vi "imp_test_v1.vi"() -> ()   [LabVIEW 2014]
uses:
  <vilib>/LabVIEW Targets/FPGA/cRIO/shared/nicrio_ModuleControls/nicrio_cRIO-9237_DataRatesRing.ctl
  <vilib>/LabVIEW Targets/FPGA/cRIO/shared/nicrio_ModuleControls/nicrio_cRIO-9237_ExcitationVoltageRing.ctl
  <vilib>/rvi/FXPMathLib/FxpSinAndCos/subVIs/nifxpmath_SinAndCos_SimConfig.ctl
  <vilib>/Platform/TimedLoop/XDataNode/timing_clust.ctl
  <vilib>/Platform/TimedLoop/XDataNode/nitl_modes.ctl
  <vilib>/Platform/TimedLoop/XDataNode/wakeup.ctl
  <vilib>/rvi/FXPMathLib/basic elements/FxpIntAccumulator/subVIs/nifxpmath_IntAccumulator_SimConfig.ctl
  <vilib>/rvi/FXPMathLib/FxpSqrt/subVIs/nifxpmath_Sqrt_SimConfig.ctl
  <vilib>/fxp/LVFixedPointOverflowPolicyTypeDef.ctl
  <vilib>/rvi/Emulation/niFpgaGetClockAttributes.vi
  <vilib>/rvi/Emulation/niFpgaSctlEmulationGetInTimedLoop.vi
  <vilib>/rvi/Emulation/niFpgaEmulationReportErrorSimple.vi
  <vilib>/rvi/Emulation/niFpgaProcessEmulError.vi
  <vilib>/rvi/interface/RandomDataEmulation/nirviRandomDataMultiElementFPGAFIFO.vi
  <instcachedir>/0/nirviRandomDataMultiElementFPGAFIFO_AD0CFC12EF974623A9C2E4184BC062B2.lvgen/nirviRandomDataMultiElementFPGAFIFO_AD0CFC12EF974623A9C2E4184BC062B2_023.vi
  <vilib>/rvi/interface/RandomDataEmulation/niFpgaRandomDataHandleErrors.vi
  <vilib>/rvi/Emulation/niFpgaCriticalErrorInLSC.vi
  <vilib>/rvi/eio/common/nirviEmuTemplateMethod_errors.vi
  <vilib>/rvi/FXPMathLib/FxpSinAndCos/simVIs/DllFxpSinAndCosTemp_sub.vi
  <vilib>/rvi/eio/common/nirviEmuTemplatePropertySet_errors.vi
  <vilib>/rvi/Analysis/common/codeGenErrors/XNode/niFpgaXNodeCodeGenErrorHandle.vi
  <vilib>/rvi/FXPMathLib/basic elements/FxpIntAccumulator/simVIs/DllFxpIntAccumulator_sub.vi
  <vilib>/rvi/FXPMathLib/FxpSqrt/simVIs/DllSqrtTemp_sub.vi
  <vilib>/rvi/DataTransferAndStorage/Container/XNode/niFpgaContainer.xnode
  <vilib>/rvi/interface/RandomDataEmulation/nirviRandomDataFpgaMultiElementTemplate.vi
  <vilib>/eio/EIONode/EIONode.xnode
  <vilib>/rvi/FXPMathLib/FxpMul/XNode/nifxpmath_Multiplier.xnode
  <vilib>/rvi/FXPMathLib/FxpSinAndCos/XNode/nifxpmath_SinAndCos.xnode
  <vilib>/rvi/Analysis/measure/butterworth/XNode/niFpgaButterworthFilter.xnode
  <vilib>/rvi/FXPMathLib/FxpSub/XNode/nifxpmath_Sub.xnode
  <vilib>/rvi/FXPMathLib/FxpAdd/XNode/nifxpmath_Add.xnode
  <vilib>/eio/EIOPropertyNode/EIOPropertyNode.xnode
  <vilib>/rvi/Analysis/measure/dc-rms/XNode/niFpgaDC-RMS.xnode
  <vilib>/Platform/TimedLoop/XDataNode/XDataNode.xnode
  <vilib>/rvi/FXPMathLib/basic elements/FxpIntAccumulator/XNode/nifxpmath_IntAccumulator.xnode
  <vilib>/rvi/FXPMathLib/FxpSqrt/XNode/nifxpmath_Sqrt.xnode
  <vilib>/rvi/eio/common/nirviEmuTemplatePropertyGet_errors.vi
  <vilib>/rvi/eio/common/nirviEmuTemplatePropertyGet_noerrors.vi
  <vilib>/rvi/eio/common/nirviEmuTemplatePropertySet_noerrors.vi
  <vilib>/Platform/TimedLoop/XDataNode/XDNodeRunTimeDep.lvlib
  <vilib>/rvi/FXPMathLib/sim/FxpSim.dll
panel:
  in  "ft_d or dt_d2":i16(ring) items=["ft_d", "ft_d2"]
  out "vb":fxp<+/-,38,8>
  out "va":fxp<+/-,38,8>
  out "ft_d2":fxp<+/-,64,59>
  out "Force_r":fxp<+/-,64,42>
  in  "Bv":fxp<+/-,22,8>
  out "D_error_dd":fxp<+/-,64,49>
  out "D_error_d":fxp<+/-,33,10>
  in  "Kv":fxp<+/-,22,8>
  out "D_error":fxp<+/-,64,33>
  out "Dr_sin_dd":fxp<+/-,64,48>
  out "Dr_sin_d":fxp<+/-,64,17>
  out "Sin omega":fxp<+/-,52,9>
  out "Dr_sin":fxp<+/-,39,10>
  in  "Sin offset":fxp<+/-,38,9>
  in  "Sin magnitude":fxp<+/-,22,7>
  out "Time now(s)":fxp<+,52,14>
  in  "Sin wave freq. (Hz)":fxp<+/-,32,6>
  in  "Dr":fxp<+/-,22,7>
  in  "Drive mode":i16(ring) items=["Backward", "Forward"]
  in  "ft_d coeff.":i32[](array[numeric])=[946630756, 63555534]
  out "ft_d":fxp<+/-,36,25>
  out "D_dd":fxp<+/-,36,24>
  in  "D_dd coeff.":i32[](array[numeric])=[946630756, 63555534]
  out "dF_PID":fxp<+/-,36,33>
  in  "dF_PID coeff.":i32[](array[numeric])=[946630756, 63555534]
  out "ft_i":fxp<+/-,34,18>
  out "F_PID":fxp<+/-,51,14>
  in  "f_tolorance":fxp<+,22,6>
  in  "Ki":fxp<+/-,36,9>
  in  "Kd":fxp<+/-,36,9>
  out "f_tilde":fxp<+/-,33,11>
  in  "Kp":fxp<+/-,36,9>
  out "vq_F":fxp<+/-,20,5> format="%.57g"
  out "vd_F":fxp<+/-,20,5>
  in  "dF_add":bool
  out "D_d(mm/s)":fxp<+/-,41,10>
  out "omega(rad/s)":fxp<+/-,20,9>
  in  "Veolcity Estimation":i16(ring) items=["T method", "M_avg method", "M method"]
  in  "Stop motor":bool
  out "D_d(T)":fxp<+/-,41,10>
  out "omega(T)":fxp<+/-,20,9>
  in  "mt0_omega":u32
  out "mt_omega":u32
  out "rad(NrTheta)":fxp<+/-,33,10>
  out "D(mm)":fxp<+/-,32,10>
  out "Encoder Position":i32
  in  "Encoder reset":bool
  in  "Ini coe.":bool
  out "Loop rate (kHz)":fxp<+/-,36,7>
  out "Strain (RMS)":fxp<+,32,44>
  in  "Strain filter coeff.":i32[](array[numeric])=[-850883994, 1909449570, 3794062, -975456236, 2033039520, 4039635]
  out "Force":fxp<+/-,32,10>
  out "Strain":fxp<+/-,42,8>
  out "Fileterd data":fxp<+/-,32,4>
  out "Raw Force":fxp<+/-,32,10>
  in  "S/F coeff":fxp<+/-,41,4>
  out "Raw Strain":fxp<+/-,42,8>
  in  "Reset":bool
  in  "Stop (Strain)":bool
  out "Mod6/AI2":fxp<+/-,32,4>
  in  "Shunt Cal Enable":bool
  in  "Half-Bridge Enable":bool
  in  "Excitation Voltage":T1 items=["2.5 Volts", "3.3 Volts", "5.0 Volts", "10.0 Volts", "External Excitation"]
  in  "Data Rate":T2=1 items=["50.000 kS/s (NI 9237)"=1, "25.000 kS/s (NI 9237)"=2, "16.667 kS/s (NI 9237)"=3, "12.500 kS/s (NI 9237)"=4, "10.000 kS/s (NI 9237)"=5, "8.333 kS/s (NI 9237)"=6, "7.143 kS/s (NI 9237)"=7, "6.250 kS/s (NI 9237)"=8, "5.556 kS/s (NI 9237)"=9, "5.000 kS/s (NI 9237)"=10, "4.545 kS/s (NI 9237)"=11, "4.167 kS/s (NI 9237)"=12, "3.846 kS/s (NI 9237)"=13, "3.571 kS/s (NI 9237)"=14, "3.333 kS/s (NI 9237)"=15, "3.125 kS/s (NI 9237)"=16, "2.941 kS/s (NI 9237)"=17, "2.778 kS/s (NI 9237)"=18, "2.632 kS/s (NI 9237)"=19, "2.500 kS/s (NI 9237)"=20, "2.381 kS/s (NI 9237)"=21, "2.273 kS/s (NI 9237)"=22, "2.174 kS/s (NI 9237)"=23, "2.083 kS/s (NI 9237)"=24, "2.000 kS/s (NI 9237)"=25, "1.923 kS/s (NI 9237)"=26, "1.852 kS/s (NI 9237)"=27, "1.786 kS/s (NI 9237)"=28, "1.724 kS/s (NI 9237)"=29, "1.667 kS/s (NI 9237)"=30, "1.613 kS/s (NI 9237)"=31]
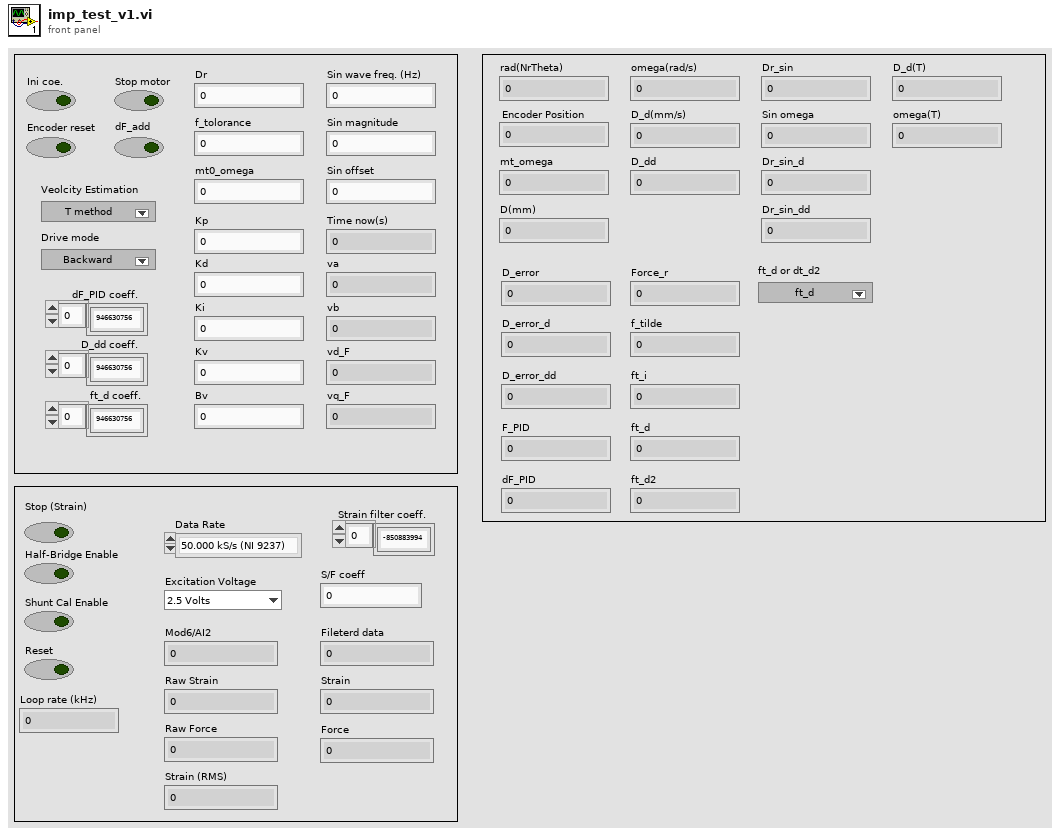
[diagram p1: front panel]
types:
  T1 = typedef "nicrio_cRIO-9237_ExcitationVoltageRing.ctl" = u8
  T2 = typedef "nicrio_cRIO-9237_DataRatesRing.ctl" = u8
  T3 = typedef "XDNodeRunTimeDep.lvlib/timing_clust.ctl" = cluster{"Expected End [f-1]":u64, "Actual End [f-1]":u64, "Finished Late? [f-1]":bool, "Expected End [i-1]":u64, "Actual End [i-1]":u64, "Finished Late? [i-1]":bool, "Expected Start [i]":u64, "Actual Start [i]":u64, "Expected Start [f]":u64, "Actual Start [f]":u64, "Source Name":string, "Structure Name":string, "Period":i64, "Deadline":i64, "Offset":i64, "Start":i64, "Priority":i32, "Timeout":i32, "Mode":T4, "Wakeup Reason":T5, "Error":errorcluster, "Source Type":string, "Secondary Source Type":string, "Global End Time":u64, "Global Start Time":u64, "Frame Duration":u64, "Iteration Duration":u64, "Assigned CPU":i32, "I/O Scan Engine Mode":u32}
  T4 = typedef "XDNodeRunTimeDep.lvlib/nitl_modes.ctl" = enum32{"No Change", "Process missed periods, maintain original phase", "Discard missed periods, maintain original phase", "Process missed periods, ignore original phase", "Discard missed periods, ignore original phase"}
  T5 = typedef "XDNodeRunTimeDep.lvlib/wakeup.ctl" = enum32{"Normal", "Aborted", "Asynchronous wakeup", "Timing source error", "Timed loop error", "Timeout"}
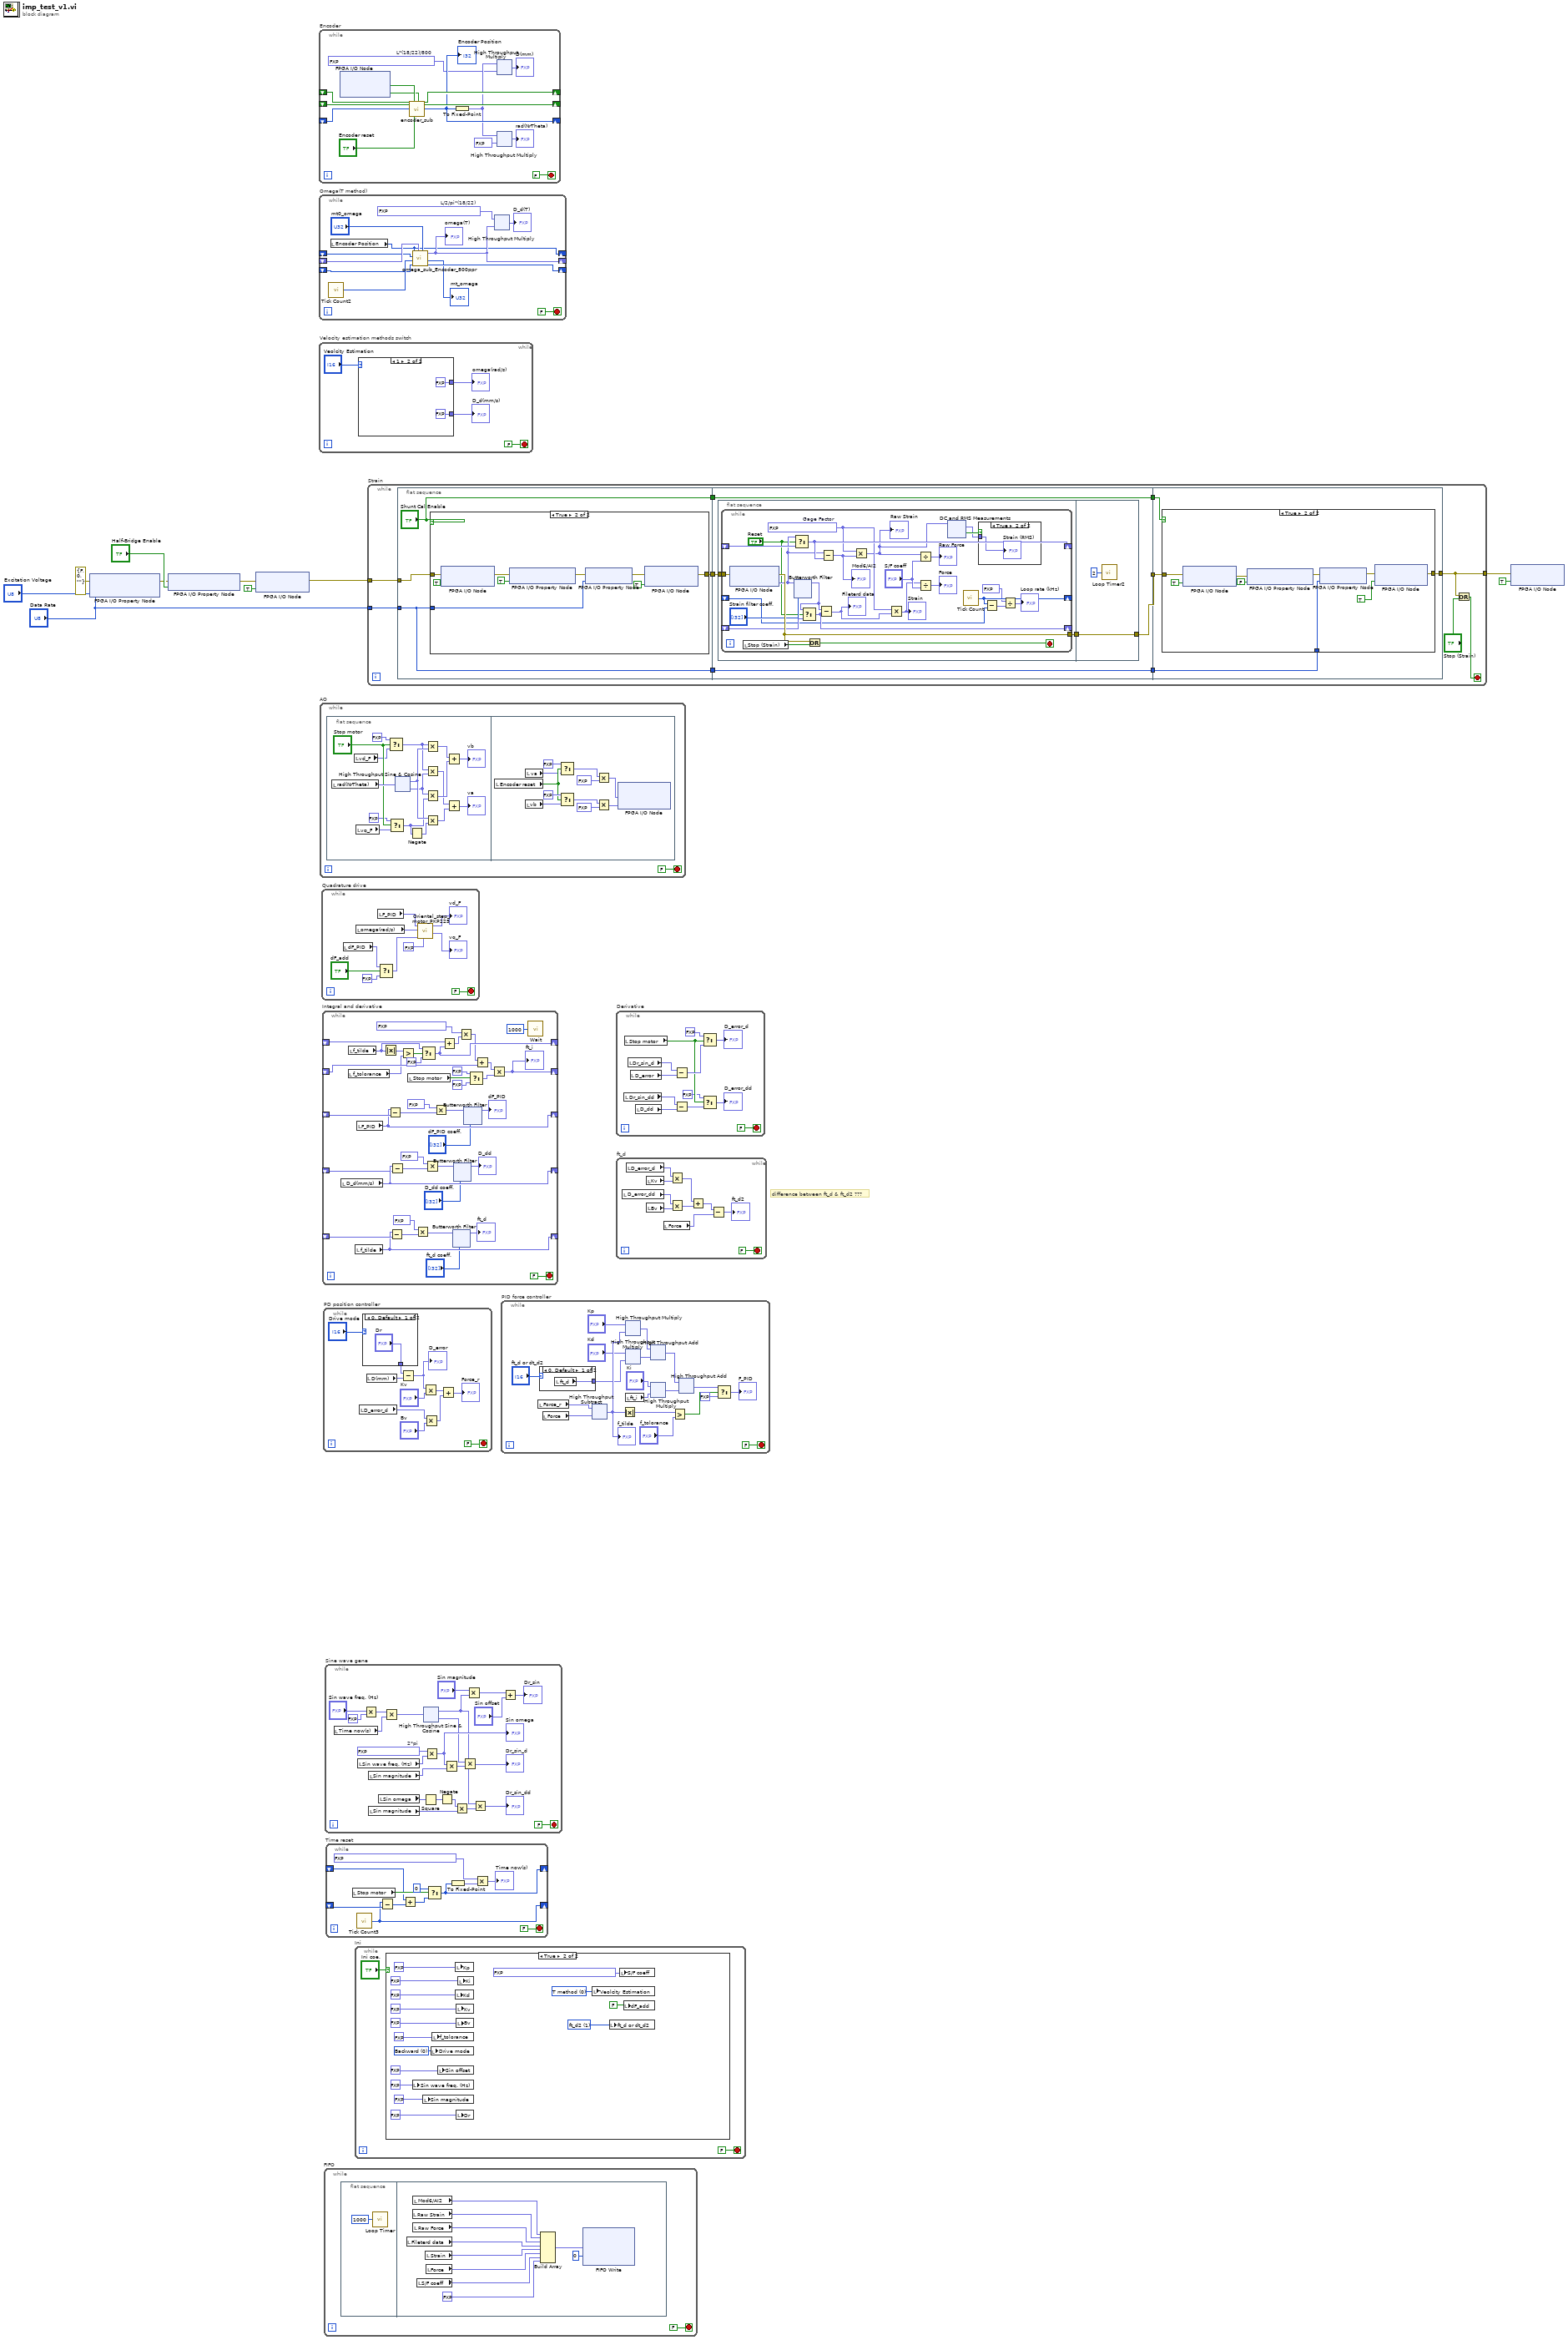
[diagram p0: block diagram]
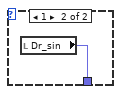
[diagram p2: hidden frame]
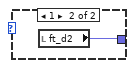
[diagram p3: hidden frame]
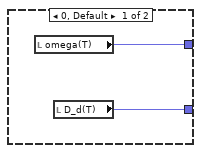
[diagram p4: hidden frame]
diagram:
  # "difference between ft_d & ft_d2 ???"
  n1 = xnode "FPGA I/O Property Node"("error in"=errorcluster {"status"=FALSE, "code"=0, "source"=""}, "Data Rate"="Data Rate", "Excitation Voltage"="Excitation Voltage") -> ("error out"=w7:errorcluster)  [unwired: 1 in, 1 out]
  n2 = xnode "FPGA I/O Property Node"("error in"=w7, "Half-Bridge Enable"="Half-Bridge Enable") -> ("error out"=w6:errorcluster)  [unwired: 1 in, 1 out]
  n3 = xnode "FPGA I/O Node"("error in"=w6, "Mod6/Start"=TRUE) -> ("error out"=w4:errorcluster)  [unwired: 1 in, 1 out]
  n4 = while "Encoder" {
    shift-right: [w22] -> _
    shift-left: _ -> [w23]
    shift-right: [w24] -> _
    shift-left: _ -> [w25]
    shift-right: [w17] -> _
    shift-left: _ -> [w21]
    stop <- FALSE stop-if-true
    w14 = fxp<+/-,32,0> 0.0020454544574022293  # L*(18/22)/800
    n5 = xnode "FPGA I/O Node"() -> ("Mod4/DI3"=w20:bool, "Mod4/DI4"=w19:bool)  [unwired: 2 in, 2 out]
    n6 = call "encoder_sub.vi"("A_pre"=w23, "B_pre"=w25, "Encoder Position_pre"=w21, "A input"=w20, "Encoder Position Reset"="Encoder reset", "B input"=w19) -> ("A"=w22:bool, "B"=w24:bool, "Encoder Position (Counts)"=w17:i32)  [unwired: 19 in]
    "Encoder Position" <- w17
    n7 = To Fixed-Point(number=w17) -> (fixed-point=w16:fxp<+/-,32,32>)  [unwired: 1 in]
    n8 = xnode ("High Throughput Multiply")("x"=w16, "y"=w14) -> ("x*y"=→"D(mm)":fxp<+/-,64,32>)
    n9 = xnode ("High Throughput Multiply")("x"=w16, "y"=fxp<+/-,16,1> 0.125) -> ("x*y"=→"rad(NrTheta)":fxp<+/-,48,33>)
  }
  n10 = while "Omega(T method)" {
    shift-right: [w27] -> _
    shift-left: _ -> [w28]
    shift-right: [w31] -> _
    shift-left: _ -> [w33]
    shift-right: [w35] -> _
    shift-left: _ -> [w36]
    stop <- FALSE stop-if-true
    w30 = fxp<+/-,32,0> 0.2604353614151478  # L/2/pi*(18/22)
    n11 = call "Tick Count2"() -> ("Tick Count(Ticks)"=w37:u32)
    n12 = local read "Encoder Position"() -> (w27:i32)
    n13 = call "omega_sub_Encoder_800ppr.vi"("mt0"="mt0_omega", "omega_pre"=w33, "ticks_m_pre"=w36, "ticks"=w37, "count_pre"=w28, "count"=w27) -> ("ticks_m"=w35:u32, "mt"=→"mt_omega":u32, "omega"=w31:fxp<+/-,20,9>)  [unwired: 3 in]
    "omega(T)" <- w31
    n14 = xnode ("High Throughput Multiply")("x"=w30, "y"=w31) -> ("x*y"=→"D_d(T)":fxp<+/-,52,9>)
  }
  n15 = while "Velocity estimation methods switch" {
    stop <- FALSE stop-if-true
    n16 = case shown="1" "Veolcity Estimation" {
      tunnel: [w43 fxp<+/-,20,9> 0.0 ("omega(T)")] -> w40
      tunnel: [w42 fxp<+/-,41,10> 0.0 ("D_d(T)")] -> w39
      frame 0, Default {
        n17 = local read "omega(T)"() -> (w43:fxp<+/-,20,9>)
        n18 = local read "D_d(T)"() -> (w42:fxp<+/-,41,10>)
      }
      frame 1 {
      }
    }
    "omega(rad/s)" <- w40
    "D_d(mm/s)" <- w39
  }
  n19 = while "AO" {
    stop <- FALSE stop-if-true
    n20 = flat-sequence {
      frame #0 {
        n21 = local read "rad(NrTheta)"() -> (w63:fxp<+/-,33,10>)
        n22 = local read "vd_F"() -> (w61:fxp<+/-,20,5>)
        n23 = local read "vq_F"() -> (w60:fxp<+/-,20,5>)
        n24 = Select(t=fxp<+/-,20,5> 0.0, s="Stop motor", f=w61) -> (s? t:f=w55:fxp<+/-,20,5>)
        n25 = Select(t=fxp<+/-,20,5> 0.0, s="Stop motor", f=w60) -> (s? t:f=w54:fxp<+/-,20,5>)
        n26 = xnode "High Throughput Sine & Cosine"("x (pi)"=w63) -> ("sin(x)"=w57:fxp<+/-,17,2>, "cos(x)"=w56:fxp<+/-,17,2>)
        n27 = Negate(x=w54) -> (-x=w53:fxp<+/-,21,6>)
        n28 = Multiply(x=w55, y=w57) -> (x*y=w52:fxp<+/-,37,7>)
        n29 = Multiply(x=w55, y=w56) -> (x*y=w50:fxp<+/-,37,7>)
        n30 = Multiply(x=w56, y=w54) -> (x*y=w51:fxp<+/-,37,7>)
        n31 = Multiply(x=w57, y=w53) -> (x*y=w49:fxp<+/-,36,6>)
        n32 = Add(x=w52, y=w51) -> (x+y=→"vb":fxp<+/-,38,8>)
        n33 = Add(x=w50, y=w49) -> (x+y=→"va":fxp<+/-,37,7>)
      }
      frame #1 {
        n34 = local read "Encoder reset"() -> (w96:bool)
        n35 = local read "vb"() -> (w94:fxp<+/-,38,8>)
        n36 = local read "va"() -> (w95:fxp<+/-,38,8>)
        n37 = Select(t=fxp<+,2,2> 3.0, s=w96, f=w95) -> (s? t:f=w100:fxp<+/-,38,8>)
        n38 = Select(t=fxp<+,1,1> 0.0, s=w96, f=w94) -> (s? t:f=w99:fxp<+/-,38,8>)
        n39 = Multiply(x=w100, y=fxp<+/-,1,0> -0.5) -> (x*y=w103:fxp<+/-,39,8>)
        n40 = Multiply(x=w99, y=fxp<+/-,1,0> -0.5) -> (x*y=w104:fxp<+/-,37,6>)
        n41 = xnode "FPGA I/O Node"("Mod8/AO2"=w103, "Mod8/AO3"=w104) -> ()  [unwired: 2 in, 2 out]
      }
    }
  }
  n42 = while "Quadrature drive" {
    stop <- FALSE stop-if-true
    n43 = local read "dF_PID"() -> (w106:fxp<+/-,36,33>)
    n44 = local read "omega(rad/s)"() -> (w114:fxp<+/-,20,9>)
    n45 = local read "F_PID"() -> (w107:fxp<+/-,51,14>)
    n46 = Select(t=w106, s="dF_add", f=fxp<+,1,1> 0.0) -> (s? t:f=w110:fxp<+/-,36,33>)
    n47 = call "Oriental_step_motor_PKP225.vi"("F_Threshold"=fxp<+,12,12> 10.0, "dFmr"=w110, "omega"=w114, "Fmr"=w107) -> ("vq_F"=→"vq_F":fxp<+/-,20,5>, "vd_F"=→"vd_F":fxp<+/-,20,5>)  [unwired: 6 in]
  }
  n48 = while "Integral and derivative" {
    shift-right: [w146] -> _
    shift-left: _ -> [w145]
    shift-right: [w138] -> _
    shift-left: _ -> [w137]
    shift-right: [w148] -> _
    shift-left: _ -> [w149]
    shift-right: [w128] -> _
    shift-left: _ -> [w127]
    shift-right: [w120] -> _
    shift-left: _ -> [w124]
    stop <- FALSE stop-if-true
    n49 = local read "D_d(mm/s)"() -> (w128:fxp<+/-,41,10>)
    n50 = local read "f_tolorance"() -> (w116:fxp<+,22,6>)
    n51 = local read "f_tilde"() -> (w150:fxp<+/-,33,11>)
    n52 = local read "f_tilde"() -> (w120:fxp<+/-,33,11>)
    n53 = local read "F_PID"() -> (w148:fxp<+/-,51,14>)
    n54 = Absolute Value(x=w150) -> (abs(x)=w152:fxp<+,33,11>)
    n55 = Subtract(x=w148, y=w149) -> (x-y=w136:fxp<+/-,52,15>)
    n56 = Subtract(x=w120, y=w124) -> (x-y=w123:fxp<+/-,34,12>)
    n57 = Subtract(x=w128, y=w127) -> (x-y=w130:fxp<+/-,42,11>)
    n58 = Greater?(x=w152, y=w116) -> (0:w153:bool)
    n59 = local read "Stop motor"() -> (w139:bool)
    n60 = Multiply(x=fxp<+/-,33,11> 1000.0, y=w123) -> (x*y=w121:fxp<+/-,64,22>)
    n61 = Select(t=w150, s=w153, f=fxp<+/-,33,11> 0.0) -> (s? t:f=w146:fxp<+/-,33,11>)
    n62 = Multiply(x=fxp<+,7,10> 1000.0, y=w130) -> (x*y=w129:fxp<+/-,49,21>)
    n63 = Multiply(x=fxp<+/-,52,15> 1000.0, y=w136) -> (x*y=w133:fxp<+/-,64,29>)
    n64 = Add(x=w145, y=w146) -> (x+y=w151:fxp<+/-,34,12>)
    n65 = xnode "Butterworth Filter"("input data"=w121, "scaled coefficients"="ft_d coeff.") -> ("output data"=→"ft_d":fxp<+/-,36,26>)  [unwired: 1 in]
    n66 = xnode "Butterworth Filter"("input data"=w129, "scaled coefficients"="D_dd coeff.") -> ("output data"=→"D_dd":fxp<+/-,36,25>)  [unwired: 1 in]
    n67 = Multiply(x=fxp<+/-,30,12> 0.000499725341796875, y=w151) -> (x*y=w144:fxp<+/-,64,24>)
    n68 = xnode "Butterworth Filter"("input data"=w133, "scaled coefficients"="dF_PID coeff.") -> ("output data"=→"dF_PID":fxp<+/-,36,33>)  [unwired: 1 in]
    n69 = Select(t=fxp<+,1,1> 0.0, s=w139, f=fxp<+,1,1> 1.0) -> (s? t:f=w142:fxp<+,1,1>)
    n70 = Add(x=w144, y=w137) -> (x+y=w143:fxp<+/-,64,24>)
    n71 = Multiply(x=w143, y=w142) -> (x*y=w138:fxp<+/-,34,18>)
    "ft_i" <- w138
    n72 = call "Wait"("Count(uSec)"=u32 1000) -> ()  [unwired: 1 out]
  }
  n73 = while "PD position controller" {
    stop <- FALSE stop-if-true
    n74 = local read "D_error_d"() -> (w182:fxp<+/-,33,10>)
    n75 = case shown="0, Default" "Drive mode" {
      tunnel: ["Dr" w191] -> w187
      frame 0, Default {
      }
      frame 1 {
        n76 = local read "Dr_sin"() -> (w191:fxp<+/-,39,10>)
      }
    }
    n77 = local read "D(mm)"() -> (w188:fxp<+/-,32,10>)
    n78 = Subtract(x=w187, y=w188) -> (x-y=w186:fxp<+/-,40,11>)
    "D_error" <- w186
    n79 = Multiply(x=w186, y="Kv") -> (x*y=w184:fxp<+/-,61,18>)
    n80 = Multiply(x=w182, y="Bv") -> (x*y=w181:fxp<+/-,55,18>)
    n81 = Add(x=w184, y=w181) -> (x+y=→"Force_r":fxp<+/-,62,19>)
  }
  n82 = while "FIFO" {
    stop <- FALSE stop-if-true
    n83 = flat-sequence {
      frame #0 {
        n84 = call "Loop Timer"("Count(uSec)"=u32 1000) -> ()  [unwired: 1 out]
      }
      frame #1 {
        n85 = local read "Fileterd data"() -> (w200:fxp<+/-,32,4>)
        n86 = local read "Raw Strain"() -> (w202:fxp<+/-,42,8>)
        n87 = local read "Mod6/AI2"() -> (w203:fxp<+/-,32,4>)
        n88 = local read "Raw Force"() -> (w201:fxp<+/-,32,10>)
        n89 = local read "S/F coeff"() -> (w197:fxp<+/-,41,4>)
        n90 = local read "Strain"() -> (w199:fxp<+/-,42,8>)
        n91 = local read "Force"() -> (w198:fxp<+/-,32,10>)
        n92 = Build Array(w203, w202, w201, w200, w199, w198, w197, fxp<+,1,1> 0.0) -> (w195:fxp<+/-,47,10>[])
        n93 = xnode ("FIFO Write")("Element"=w195, "Timeout"=0) -> ()  [unwired: 1 in, 2 out]
      }
    }
  }
  n94 = while "Sine wave gene" {
    stop <- FALSE stop-if-true
    w218 = fxp<+,20,3> 6.2831878662109375  # 2*pi
    n95 = local read "Time now(s)"() -> (w224:fxp<+,52,14>)
    n96 = local read "Sin wave freq. (Hz)"() -> (w217:fxp<+/-,32,6>)
    n97 = Multiply(x="Sin wave freq. (Hz)", y=fxp<+/-,32,6> 2.0) -> (x*y=w225:fxp<+/-,64,12>)
    n98 = local read "Sin magnitude"() -> (w215:fxp<+/-,22,7>)
    n99 = local read "Sin magnitude"() -> (w208:fxp<+/-,22,7>)
    n100 = local read "Sin omega"() -> (w211:fxp<+/-,52,9>)
    n101 = Multiply(x=w225, y=w224) -> (x*y=w223:fxp<+/-,64,25>)
    n102 = Square(x=w211) -> (x^2=w210:fxp<+,64,16>)
    n103 = xnode "High Throughput Sine & Cosine"("x (pi)"=w223) -> ("sin(x)"=w205:fxp<+/-,16,2>, "cos(x)"=w213:fxp<+/-,16,2>)
    n104 = Multiply(x=w218, y=w217) -> (x*y=w216:fxp<+/-,52,9>)
    "Sin omega" <- w216
    n105 = Negate(x=w210) -> (-x=w209:fxp<+/-,64,17>)
    n106 = Multiply(x=w216, y=w215) -> (x*y=w214:fxp<+/-,64,15>)
    n107 = Multiply(x=w209, y=w208) -> (x*y=w207:fxp<+/-,64,24>)
    n108 = Multiply(x=w213, y=w214) -> (x*y=→"Dr_sin_d":fxp<+/-,64,17>)
    n109 = Multiply(x="Sin magnitude", y=w205) -> (x*y=w221:fxp<+/-,38,9>)
    n110 = Multiply(x=w205, y=w207) -> (x*y=→"Dr_sin_dd":fxp<+/-,64,26>)
    n111 = Add(x=w221, y="Sin offset") -> (x+y=→"Dr_sin":fxp<+/-,39,10>)
  }
  n112 = while "Time reset" {
    shift-right: [w267] -> _
    shift-left: _ -> [w268]
    shift-right: [w262] -> _
    shift-left: _ -> [w263]
    stop <- FALSE stop-if-true
    n113 = local read "Stop motor"() -> (w269:bool)
    n114 = call "Tick Count3"() -> ("Tick Count(uSec)"=w267:u32)
    n115 = Subtract(x=w267, y=w268) -> (x-y=w266:u32)
    n116 = Add(x=w263, y=w266) -> (x+y=w265:u32)
    n117 = Select(t=u32 0, s=w269, f=w265) -> (s? t:f=w262:u32)
    n118 = To Fixed-Point(number=w262) -> (fixed-point=w261:fxp<+,32,32>)  [unwired: 1 in]
    n119 = Multiply(x=fxp<+,20,-18> 1.0000003385357559e-06, y=w261) -> (x*y=→"Time now(s)":fxp<+,52,14>)
  }
  n120 = while "Ini" {
    stop <- FALSE stop-if-true
    n121 = case shown="True" "Ini coe." {
      frame False {
      }
      frame True {
        w272 = i16 1 items=["ft_d", "ft_d2"] ("ft_d or dt_d2")
        w278 = i16 0 items=["T method", "M_avg method", "M method"] ("Veolcity Estimation")
        w280 = i16 0 items=["Backward", "Forward"] ("Drive mode")
        n122 = local write "Sin wave freq. (Hz)"(fxp<+/-,32,6> 1.0 ("Sin wave freq. (Hz)")) -> ()
        n123 = local write "Sin magnitude"(fxp<+/-,22,7> 10.0 ("Sin magnitude")) -> ()
        n124 = local write "Drive mode"(w280) -> ()
        n125 = local write "f_tolorance"(fxp<+,22,6> 10.0 ("f_tolorance")) -> ()
        n126 = local write "Sin offset"(fxp<+/-,38,9> 0.0 ("Sin offset")) -> ()
        n127 = local write "Kp"(fxp<+/-,36,9> 50.0 ("Kp")) -> ()
        n128 = local write "Kd"(fxp<+/-,36,9> 0.0 ("Kd")) -> ()
        n129 = local write "Kv"(fxp<+/-,22,8> 1.0 ("Kv")) -> ()
        n130 = local write "Bv"(fxp<+/-,22,8> 0.0 ("Bv")) -> ()
        n131 = local write "Dr"(fxp<+/-,22,7> 0.0 ("Dr")) -> ()
        n132 = local write "Ki"(fxp<+/-,36,9> 0.0 ("Ki")) -> ()
        n133 = local write "Veolcity Estimation"(w278) -> ()
        n134 = local write "ft_d or dt_d2"(w272) -> ()
        n135 = local write "S/F coeff"(fxp<+/-,41,4> 1.047803380060941e-06 ("S/F coeff")) -> ()
        n136 = local write "dF_add"(FALSE ("dF_add")) -> ()
      }
    }
  }
  n137 = while "Strain" {
    tunnel: w4 -> [w297]
    tunnel: "Data Rate" -> [w296]
    tunnel: [w288] -> w2
    stop <- w289 stop-if-true
    n138 = flat-sequence {
      tunnel: w297 -> [w301]
      tunnel: w296 -> [w300]
      tunnel: [w300] -> w295
      tunnel: ["Shunt Cal Enable"] -> w294
      tunnel: [w298] -> w293
      tunnel: w295 -> [w314]
      tunnel: w294 -> [w315]
      tunnel: w293 -> [w316]
      tunnel: [w315] -> w292
      tunnel: [w313] -> w291
      tunnel: [w314] -> w290
      tunnel: w292 -> [w497]
      tunnel: w291 -> [w496]
      tunnel: w290 -> [w495]
      tunnel: [w494] -> w288
      frame #0 {
        n139 = case shown="True" "Shunt Cal Enable" {
          tunnel: w301 -> [w302 w309]
          tunnel: w300 -> [_ w307]
          tunnel: [w302 w304] -> w298
          frame False {
          }
          frame True {
            n140 = xnode "FPGA I/O Node"("error in"=w309, "Mod6/Stop"=TRUE) -> ("error out"=w310:errorcluster)  [unwired: 1 in, 1 out]
            n141 = xnode "FPGA I/O Property Node"("error in"=w310, "Shunt Cal Enable"=TRUE) -> ("error out"=w308:errorcluster)  [unwired: 1 in, 1 out]
            n142 = xnode "FPGA I/O Property Node"("error in"=w308, "Data Rate"=w307) -> ("error out"=w306:errorcluster)  [unwired: 1 in, 1 out]
            n143 = xnode "FPGA I/O Node"("error in"=w306, "Mod6/Start"=TRUE) -> ("error out"=w304:errorcluster)  [unwired: 1 in, 1 out]
          }
        }
      }
      frame #1 {
        n144 = flat-sequence {
          tunnel: w316 -> [w318]
          tunnel: [w317] -> w312
          tunnel: [w493] -> w313
          tunnel: w312 -> [w493]
          frame #0 {
            n145 = while {
              tunnel: w318 -> [w345]
              tunnel: [w343] -> w317
              shift-right: [w341] -> _
              shift-left: _ -> [w342]
              shift-right: [w337] -> _
              shift-left: _ -> [w338]
              shift-right: [w324] -> _
              shift-left: _ -> [w325]
              stop <- w330 stop-if-true
              w335 = fxp<+,20,2> 2.115001678466797  # Gage Factor
              n146 = xnode "FPGA I/O Node"("error in"=w345) -> ("error out"=w343:errorcluster, "Mod6/AI2"=w339:fxp<+/-,24,-4>)  [unwired: 1 in, 1 out]
              n147 = local read "Stop (Strain)"() -> (w344:bool)
              n148 = xnode "Butterworth Filter"("input data"=w339, "scaled coefficients"="Strain filter coeff.") -> ("output data"=w336:fxp<+/-,28,0>)  [unwired: 1 in]
              n149 = Select(t=w339, s="Reset", f=w342) -> (s? t:f=w341:fxp<+/-,24,-4>)
              n150 = Select(t=w336, s="Reset", f=w338) -> (s? t:f=w337:fxp<+/-,28,0>)
              n151 = Or(x=w343, y=w344) -> (x .or. y?=w330:bool)
              n152 = Subtract(x=w336, y=w337) -> (x-y=w334:fxp<+/-,32,16>)
              "Fileterd data" <- w334
              n153 = Subtract(x=w339, y=w341) -> (x-y=w340:fxp<+/-,25,-3>)
              "Mod6/AI2" <- w340
              n154 = Multiply(x=w335, y=w340) -> (x*y=w322:fxp<+/-,41,6>)
              "Raw Strain" <- w322
              n155 = Multiply(x=w335, y=w334) -> (x*y=w332:fxp<+/-,41,6>)
              "Strain" <- w332
              n156 = Divide(x=w322, y="S/F coeff") -> (x/y=→"Raw Force":fxp<+/-,64,44>)
              n157 = Divide(x=w332, y="S/F coeff") -> (x/y=→"Force":fxp<+/-,64,44>)
              n158 = xnode ("DC and RMS Measurements")("input data"=w322) -> ("RMS"=w326:fxp<+,32,6>, "output valid"=w327:bool)  [unwired: 1 in, 1 out]
              n159 = call "Tick Count"() -> ("Tick Count(uSec)"=w324:u32)
              n160 = case shown="True" w327 {
                tunnel: w326 -> [_ w346]
                frame False {
                }
                frame True {
                  "Strain (RMS)" <- w346
                }
              }
              n161 = Subtract(x=w324, y=w325) -> (x-y=w321:fxp<+/-,32,16>)
              n162 = Divide(x=fxp<+,7,10> 1000.0, y=w321) -> (x/y=→"Loop rate (kHz)":fxp<+/-,40,27>)
            }
          }
          frame #1 {
            n163 = call "Loop Timer2"("Count(uSec)"=u32 2) -> ()  [unwired: 1 out]
          }
        }
      }
      frame #2 {
        n164 = case shown="True" w497 {
          tunnel: w496 -> [w498 w506]
          tunnel: w495 -> [_ w502]
          tunnel: [w498 w499] -> w494
          frame False {
          }
          frame True {
            n165 = xnode "FPGA I/O Node"("error in"=w506, "Mod6/Stop"=TRUE) -> ("error out"=w504:errorcluster)  [unwired: 1 in, 1 out]
            n166 = xnode "FPGA I/O Property Node"("error in"=w504, "Shunt Cal Enable"=FALSE) -> ("error out"=w503:errorcluster)  [unwired: 1 in, 1 out]
            n167 = xnode "FPGA I/O Property Node"("error in"=w503, "Data Rate"=w502) -> ("error out"=w501:errorcluster)  [unwired: 1 in, 1 out]
            n168 = xnode "FPGA I/O Node"("error in"=w501, "Mod6/Start"=TRUE) -> ("error out"=w499:errorcluster)  [unwired: 1 in, 1 out]
          }
        }
      }
    }
    n169 = Or(x=w288, y="Stop (Strain)") -> (x .or. y?=w289:bool)
  }
  n170 = while "PID force controller" {
    stop <- FALSE stop-if-true
    n171 = local read "Force_r"() -> (w512:fxp<+/-,64,42>)
    n172 = case shown="0, Default" "ft_d or dt_d2" {
      tunnel: [w528 w529] -> w508
      frame 0, Default {
        n173 = local read "ft_d"() -> (w528:fxp<+/-,36,25>)
      }
      frame 1 {
        n174 = local read "ft_d2"() -> (w529:fxp<+/-,64,59>)
      }
    }
    n175 = local read "Force"() -> (w526:fxp<+/-,32,10>)
    n176 = xnode "High Throughput Subtract"("x"=w512, "y"=w526) -> ("x-y"=w525:fxp<+/-,64,43>)
    "f_tilde" <- w525
    n177 = Absolute Value(x=w525) -> (abs(x)=w516:fxp<+,64,43>)
    n178 = local read "ft_i"() -> (w511:fxp<+/-,34,18>)
    n179 = xnode ("High Throughput Multiply")("x"="Kp", "y"=w525) -> ("x*y"=w523:fxp<+/-,64,52>)
    n180 = xnode ("High Throughput Multiply")("x"="Kd", "y"=w508) -> ("x*y"=w522:fxp<+/-,64,68>)
    n181 = xnode ("High Throughput Add")("x"=w523, "y"=w522) -> ("x+y"=w519:fxp<+/-,64,69>)
    n182 = xnode ("High Throughput Multiply")("x"="Ki", "y"=w511) -> ("x*y"=w520:fxp<+/-,64,27>)
    n183 = Greater?(x=w516, y="f_tolorance") -> (0:w514:bool)
    n184 = xnode ("High Throughput Add")("x"=w519, "y"=w520) -> ("x+y"=w518:fxp<+/-,64,70>)
    n185 = Select(t=w518, s=w514, f=fxp<+/-,51,14> 0.0) -> (s? t:f=→"F_PID":fxp<+/-,64,70>)
  }
  n186 = while "Derivative" {
    stop <- FALSE stop-if-true
    n187 = local read "Dr_sin_dd"() -> (w535:fxp<+/-,64,48>)
    n188 = local read "Stop motor"() -> (w533:bool)
    n189 = local read "Dr_sin_d"() -> (w538:fxp<+/-,64,17>)
    n190 = local read "D_error"() -> (w539:fxp<+/-,64,33>)
    n191 = local read "D_dd"() -> (w536:fxp<+/-,36,24>)
    n192 = Subtract(x=w538, y=w539) -> (x-y=w537:fxp<+/-,64,34>)
    n193 = Subtract(x=w535, y=w536) -> (x-y=w534:fxp<+/-,64,49>)
    n194 = Select(t=fxp<+,1,1> 0.0, s=w533, f=w537) -> (s? t:f=→"D_error_d":fxp<+/-,64,34>)
    n195 = Select(t=fxp<+/-,64,49> 0.0, s=w533, f=w534) -> (s? t:f=→"D_error_dd":fxp<+/-,64,49>)
  }
  n196 = while "ft_d" {
    stop <- FALSE stop-if-true
    n197 = local read "D_error_dd"() -> (w548:fxp<+/-,64,49>)
    n198 = local read "D_error_d"() -> (w550:fxp<+/-,33,10>)
    n199 = local read "Kv"() -> (w551:fxp<+/-,22,8>)
    n200 = local read "Bv"() -> (w549:fxp<+/-,22,8>)
    n201 = local read "Force"() -> (w544:fxp<+/-,32,10>)
    n202 = Multiply(x=w550, y=w551) -> (x*y=w546:fxp<+/-,55,18>)
    n203 = Multiply(x=w548, y=w549) -> (x*y=w547:fxp<+/-,64,57>)
    n204 = Add(x=w546, y=w547) -> (x+y=w545:fxp<+/-,64,58>)
    n205 = Subtract(x=w545, y=w544) -> (x-y=→"ft_d2":fxp<+/-,64,59>)
  }
  n206 = xnode "FPGA I/O Node"("error in"=w2, "Mod6/Stop"=TRUE) -> ()  [unwired: 1 in, 2 out]
